vi "add_float64.vi"   [LabVIEW 2010]
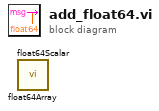
[diagram p0: block diagram]
diagram:
  n1 = call "float64Array.vi"() -> ()  [unwired: 5 in, 1 out]
  n2 = call "float64Scalar.vi"() -> ()  [unwired: 5 in, 1 out]
